vi "Load_Installer_Type.vi"(8 "error in (no error)":errorcluster, 11 "buildObject":T1) -> (0 "error out":errorcluster, 3 "Class out":refnum<class "Installer.lvclass">)   [LabVIEW 2020, in "Installer.lvclass"]
uses:
  <vilib>/AppBuilder/IB_Classes/Installer/Installer.lvclass
  <vilib>/AppBuilder/IB_Classes/Installer/Installer.lvclass/Installer.ctl
  <resource>/Framework/Providers/API/ItemRef.ctl
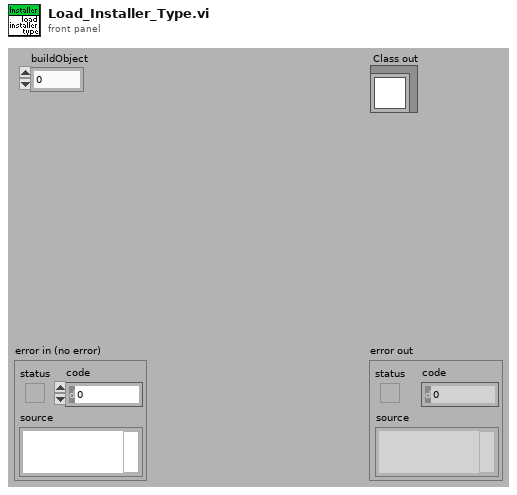
[diagram p1: front panel]
types:
  T1 = typedef "ItemRef.ctl" = u64
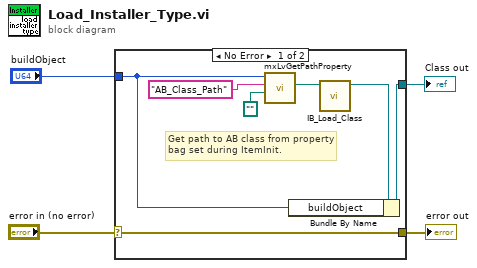
[diagram p0: block diagram]
diagram:
  n1 = case shown="No Error" "error in (no error)" {
    selector: "error in (no error)" -> [w11 w12]
    tunnel: [w11 w12] -> w3
    tunnel: [w10 _] -> w2
    tunnel: "buildObject" -> [w8 _]
    frame No Error {
      # "Get path to AB class from property bag set during ItemInit."
      n2 = call <resource>:"mxLvGetPathProperty.vi"("Default Path"=path "", "Tag"="AB_Class_Path", "Item"=w8) -> ("Path"=w7:path)  [unwired: 1 in, 7 out]
      n3 = call <vilib>:"IB_Load_Class.vi"("IB_Class path"=w7) -> ("IB_Installer out"=w9:refnum<class "Installer.lvclass">)  [unwired: 1 in, 9 out]
      n4 = Bundle By Name(cluster=w9, "buildObject"=w8) -> (w10:refnum<class "Installer.lvclass">)
    }
    frame Error {
    }
  }
  "error out" <- w3
  "Class out" <- w2
